vi "Get ControlPacket Bytes.vi"(6 "Validate? (F)":bool, 8 "error in (no error)":errorcluster, 11 "ControlPacket":refnum<class "ControlPacket.lvclass">) -> (0 "error out":errorcluster, 2 "Bytes Stream":u8[](array[numeric]) format="%08b", 3 "ControlPacket dup":refnum<class "ControlPacket.lvclass">)   [LabVIEW 2013, in "ControlPacket.lvclass"]
uses:
  ControlPacket.lvclass
  ControlPacket.lvclass/ControlPacket.ctl
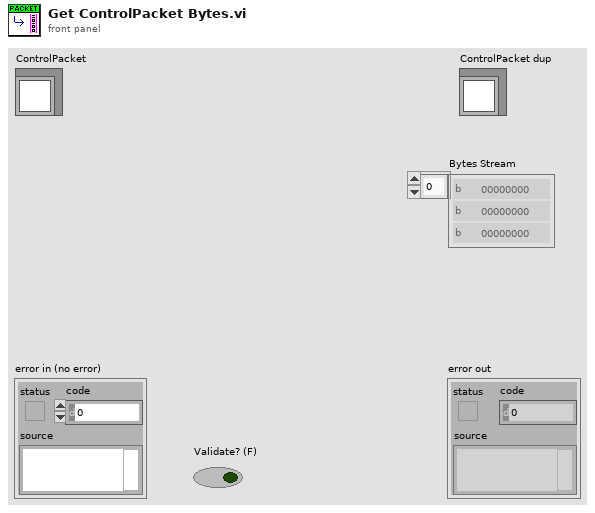
[diagram p1: front panel]
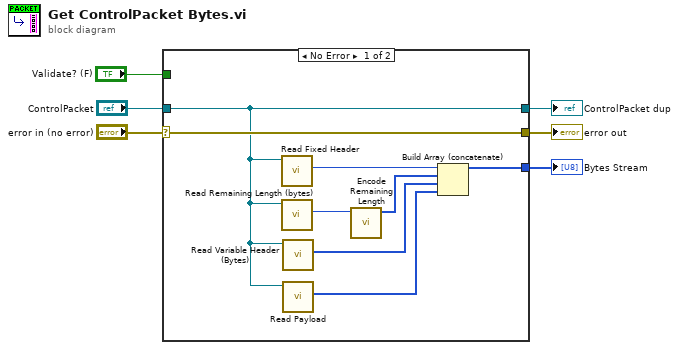
[diagram p0: block diagram]
diagram:
  n1 = case shown="No Error" "error in (no error)" {
    selector: "error in (no error)" -> [w14 w16]
    tunnel: [w14 w16] -> w5
    tunnel: [w13 w15] -> w3
    tunnel: "ControlPacket" -> [w13 w15]
    tunnel: "Validate? (F)" -> [_ _]
    tunnel: [w7 _] -> w1
    frame No Error {
      n2 = call "Read Fixed Header.vi"("ControlPacket in"=w13) -> ("Fixed Header"=w12:u8)  [unwired: 9 in, 1 out]
      n3 = call "Read Remaining Length (bytes).vi"("ControlPacket in"=w13) -> ("Remaining Length (bytes)"=w11:u32)  [unwired: 8 in, 2 out]
      n4 = call "Read Variable Header (Bytes).vi"("ControlPacket in"=w13) -> ("Variable Header (Bytes)"=w9:u8[])  [unwired: 9 in, 1 out]
      n5 = call "Read Payload.vi"("ControlPacket in"=w13) -> ("Payload"=w8:u8[])  [unwired: 9 in, 1 out]
      n6 = call "Encode Remaining Length.vi"("Remaining Length (bytes)"=w11) -> ("Encoded Remaining Length"=w10:u8[])  [unwired: 9 in, 1 out]
      n7 = Build Array (concatenate)(w12, w10, w9, w8) -> (w7:u8[])
    }
    frame Error {
    }
  }
  "error out" <- w5
  "ControlPacket dup" <- w3
  "Bytes Stream" <- w1
